vi "ProdaNG.Tree.WabcoPart.Empty.vi"(7 "Tree":refnum<vi>, 8 "error in (no error)":errorcluster, 10 "Tag":string) -> (0 "error out":errorcluster)   [LabVIEW 2016]
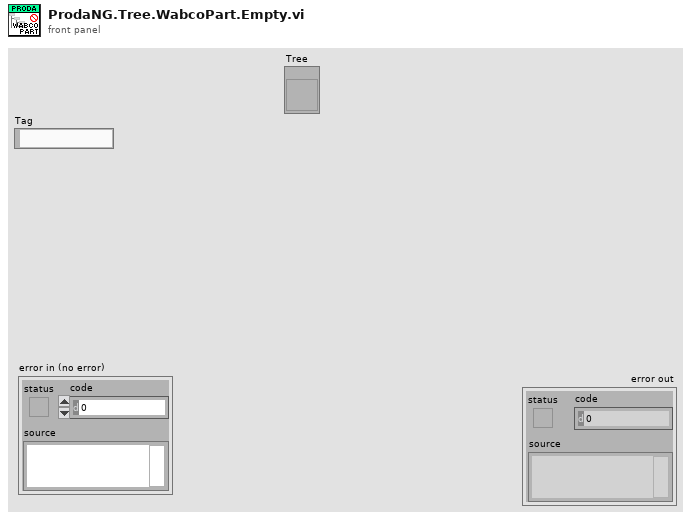
[diagram p1: front panel]
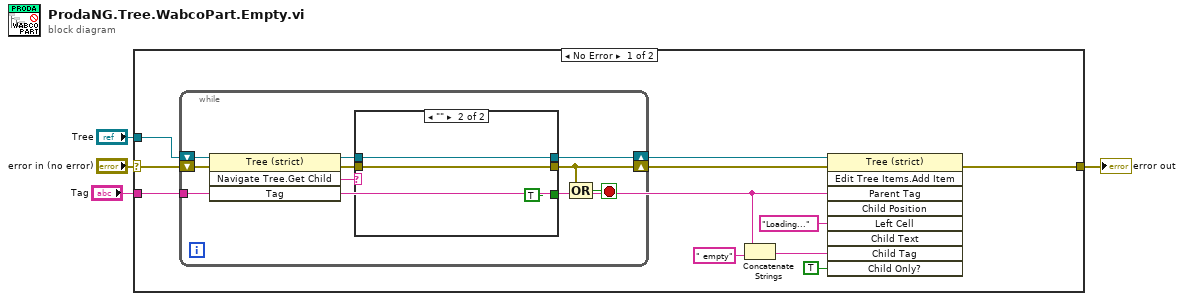
[diagram p0: block diagram]
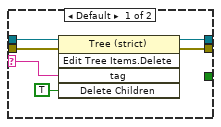
[diagram p2: hidden frame]
diagram:
  n1 = case shown="No Error" "error in (no error)" {
    selector: "error in (no error)" -> [w14 w34]
    tunnel: [w6 w34] -> w3
    tunnel: "Tree" -> [w13 _]
    tunnel: "Tag" -> [w10 _]
    frame No Error {
      n2 = while {
        shift-right: [w18] -> w11
        shift-left: w13 -> [w24]
        shift-right: [w17] -> w12
        shift-left: w14 -> [w22]
        tunnel: w10 -> [w23]
        stop <- w16 stop-if-true
        n3 = invoke class="Tree (strict)" method="Navigate Tree.Get Child"(reference=w24, error in=w22, "Tag"=w23) -> (reference out=w21:refnum<vi>, error out=w20:errorcluster, "Navigate Tree:Get Child"=w19:string)  [unwired: 1 in, 1 out]
        n4 = case shown="\"\"" w19 {
          selector: w19 -> [w28 _]
          tunnel: w21 -> [w30 w33]
          tunnel: w20 -> [w29 w32]
          tunnel: [w27 w33] -> w18
          tunnel: [w26 w32] -> w17
          tunnel: [_ TRUE] -> w15
          frame Default {
            n5 = invoke class="Tree (strict)" method="Edit Tree Items.Delete"(reference=w30, error in=w29, "tag"=w28, "Delete Children"=TRUE ("Delete Children?")) -> (reference out=w27:refnum<vi>, error out=w26:errorcluster)  [unwired: 1 in, 3 out]
          }
          frame "" {
          }
        }
        n6 = Compound Arithmetic op=OR(w17, w15) -> (w16:bool)
      }
      n7 = Concatenate Strings(w10, " empty" ("string")) -> (w8:string)
      n8 = invoke class="Tree (strict)" method="Edit Tree Items.Add Item"(reference=w11, error in=w12, "Parent Tag"=w10, "Left Cell"="Loading..." ("Left Cell String"), "Child Tag"=w8, "Child Only?"=TRUE) -> (error out=w6:errorcluster)  [unwired: 3 in, 8 out]
    }
    frame Error {
    }
  }
  "error out" <- w3
